vi "Error_ErrorLogMain.vi"() -> (10 "ErrorFilePath":path=path "c:/ErrorLogFiles/ErrorLog.txt")   [LabVIEW 2016]
panel:
  out "error out":errorcluster
  out "Iterations":i32
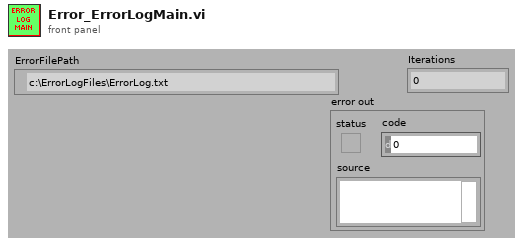
[diagram p1: front panel]
types:
  T1 = enum16{"open", "replace", "create", "open or create", "replace or create", "replace or create with confirmation"}
  T2 = cluster{"Current Path":path, "Data Files Path":path, "ASCII Files Path":path, "Error Logs Path":path, "Excel Files Path":path, "Snap-Shots Path":path, "Reports Path":path, "Support Files Path":path, "Motor Type Files":path, "Report Templates":path, "Test Sequence Files":path, "Default_VIT_Path":path, "Waterfall_VIT_Path":path, "Mimic_VIT_Path":path, "Trend_VIT_Path":path, "TestTMP1_STBR":path, "TestTMP2_MRT":path, "TestTMP3_OCCT":path, "TestTMP4_SCCT":path, "TestTMP5_ORT":path, "TestTMP6_STAR":path}
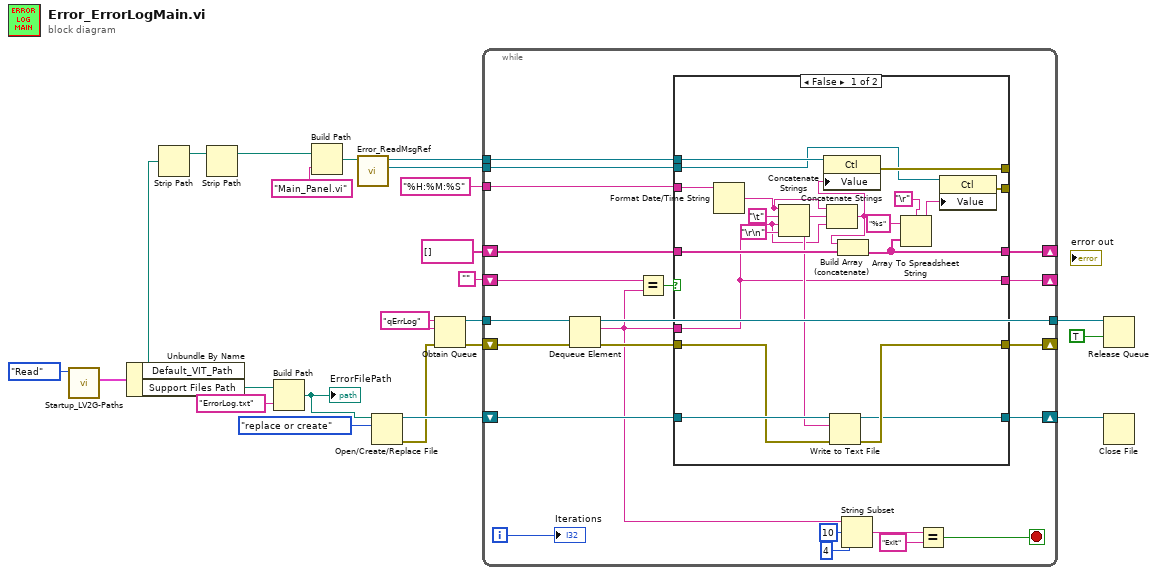
[diagram p0: block diagram]
diagram:
  w22 = "qErrLog" ("name (unnamed)")
  n1 = call "Startup_LV2G-Paths.vi"("Action"=enum16{"Read", "Write"}."Read") -> ("Paths"=w12:T2)  [unwired: 2 in, 8 out]
  n2 = Unbundle By Name(w12) -> ("Default_VIT_Path"=w8:path, "Support Files Path"=w11:path)
  n3 = Strip Path(path=w8) -> (stripped path=w2:path)  [unwired: 1 out]
  n4 = Strip Path(path=w2) -> (stripped path=w1:path)  [unwired: 1 out]
  n5 = Build Path(base path=w11, name or relative path="ErrorLog.txt") -> (appended path=w9:path)
  "ErrorFilePath" <- w9
  n6 = Build Path(base path=w1, name or relative path="Main_Panel.vi") -> (appended path=w6:path)
  n7 = call "Error_ReadMsgRef.vi"("vi path"=w6) -> ("ErrorMsgArray"=w4:refnum<vi>, "ErrorMsg"=w5:refnum<vi>)  [unwired: 1 in, 6 out]
  n8 = Open/Create/Replace File(file path (use dialog)=w9, operation (0:open)=T1."replace or create") -> (refnum out=w21:refnum<file>, error out=w20:errorcluster)  [unwired: 1 in, 4 out]
  n9 = Obtain Queue(name (unnamed)=w22, element data type=w22, error in (no error)=w20) -> (queue out=w24:refnum<queue>, error out=w23:errorcluster)  [unwired: 2 in, 1 out]
  n10 = while {
    tunnel: w24 -> [w46]
    shift-right: [w44] -> _
    shift-left: w23 -> [w40]
    shift-right: [w43] -> w17
    shift-left: w21 -> [w45]
    tunnel: "%H:%M:%S" ("time format string (%c)") -> [w42]
    tunnel: [w38] -> w16
    shift-right: [w35] -> _
    shift-left: "" ("name (unnamed)") -> [w36]
    tunnel: w5 -> [w34]
    shift-right: [w26] -> _
    shift-left: string[] [] -> [w27]
    tunnel: w4 -> [w25]
    i -> [w41]
    stop <- w28 stop-if-true
    n11 = Dequeue Element(queue=w46, error in (no error)=w40) -> (queue out=w38:refnum<queue>, element=w30:string, error out=w39:errorcluster)  [unwired: 2 out]
    n12 = Equal?(x=w36, y=w30) -> (x = y?=w37:bool)
    n13 = case shown="False" w37 {
      tunnel: w45 -> [w66 w69]
      tunnel: [w65 w70] -> w44
      tunnel: [w64 w69] -> w43
      tunnel: w42 -> [w63 _]
      tunnel: w30 -> [w49 w68]
      tunnel: w39 -> [w62 w70]
      tunnel: [w49 w68] -> w35
      tunnel: w34 -> [w60 _]
      tunnel: [w59 _] -> _
      tunnel: w27 -> [w58 w67]
      tunnel: [w54 w67] -> w26
      tunnel: w25 -> [w53 _]
      tunnel: [w52 _] -> _
      frame False {
        w50 = "\t"
        n14 = Format Date/Time String(time format string (%c)=w63) -> (date/time string=w51:string)  [unwired: 2 out]
        n15 = Concatenate Strings(w51, w50, w49, "\r\n") -> (w57:string)
        n16 = Concatenate Strings(w51, w50, w49) -> (w48:string)
        n17 = property class="Ctl"(reference=w60, "Value"=w48) -> (error out=w59:errorcluster)  [unwired: 1 in, 1 out]
        n18 = Write to Text File(file (use dialog)=w66, text=w57, error in=w62) -> (refnum out=w64:refnum<file>, error out=w65:errorcluster)  [unwired: 2 out]
        n19 = Build Array (concatenate)(w48, w58) -> (w54:string[])
        n20 = Array To Spreadsheet String(delimiter (Tab)="\r", array=w54, 3:"%s" ("format string")) -> (spreadsheet string=w56:string)
        n21 = property class="Ctl"(reference=w53, "Value"=w56) -> (error out=w52:errorcluster)  [unwired: 1 in, 1 out]
      }
      frame True {
      }
    }
    n22 = String Subset(string=w30, offset (0)=10, length (rest)=4 ("length (rest)")) -> (substring=w29:string)
    n23 = Equal?(x=w29, y="Exit") -> (x = y?=w28:bool)
    "Iterations" <- w41
  }
  n24 = Release Queue(queue=w16, force destroy? (F)=TRUE) -> ()  [unwired: 1 in, 3 out]
  n25 = Close File(refnum=w17) -> ()  [unwired: 1 in, 2 out]
